vi "Error handler_Init.vi"(0 "reference in":refnum<class "Error handler.lvclass"> caption="This control should only be used when\na sub class is inheriting this class", 3 "LoadFPOnError":bool, 5 "Error In":errorcluster, 6 "Name":string, 8 "Testing":bool) -> (14 "reference out":refnum<class "Error handler.lvclass"> caption="This indicator should only be used when\na sub class is inheriting this class", 19 "Error Out":errorcluster)   [LabVIEW 2019, in "Error handler.lvclass"]
uses:
  Error handler.lvclass
  <vilib>/Utility/sysdir.llb/System Directory Type.ctl
  ErrorLogFile_class/ErrorLogFile.lvclass
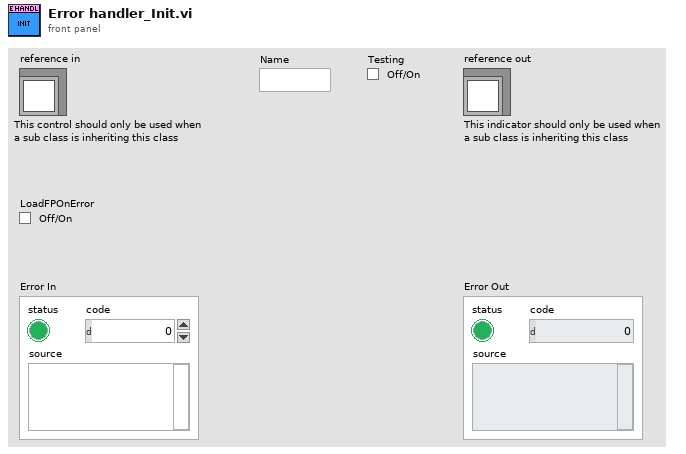
[diagram p1: front panel]
types:
  T1 = typedef "Error handler.lvclass/ObjectAttributes.ctl" = cluster{"ErrorBroadcastEvent":refnum<user-event>, "LoadFPOnError":bool, "ErrorLogFile":refnum<class "ErrorLogFile.lvclass">, "Testing":bool, "Name":string}
  T2 = typedef "System Directory Type.ctl" = i32
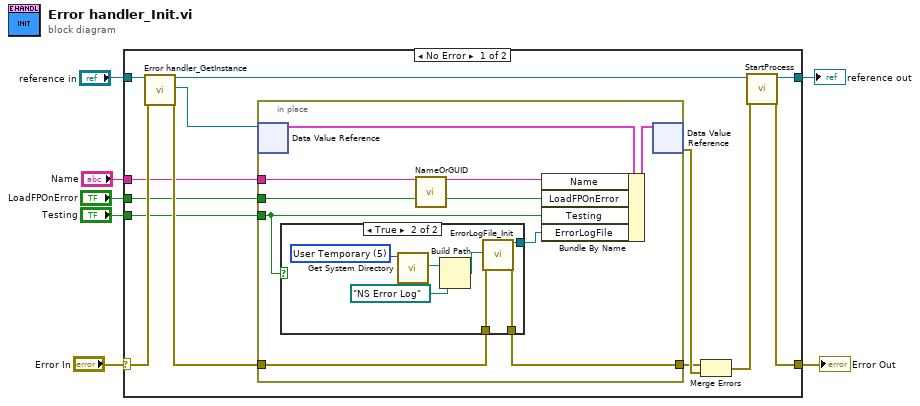
[diagram p0: block diagram]
diagram:
  n1 = case shown="No Error" "Error In" {
    selector: "Error In" -> [w19 w39]
    tunnel: [w11 w39] -> w6
    tunnel: "reference in" -> [w18 w38]
    tunnel: [w13 w38] -> w4
    tunnel: "LoadFPOnError" -> [w10 _]
    tunnel: "Testing" -> [w9 _]
    tunnel: "Name" -> [w8 _]
    frame No Error {
      n2 = call "Error handler_GetInstance.vi"("reference in"=w18, "error in"=w19) -> ("reference out"=w14:refnum<class "Error handler.lvclass">, "DVRRefOut"=w17:refnum<data-value>, "error out"=w16:errorcluster)  [unwired: 13 in, 2 out]
      n3 = in-place {
        in-place-border: w16 -> [w23]
        in-place-border: [w24] -> w15
        in-place-border: w10 -> [w27]
        in-place-border: w9 -> [w26]
        in-place-border: w8 -> [w22]
        n4 = in-place-dvr #1(w17) -> (w28:T1)  [unwired: 1 out]
        n5 = case shown="True" w26 {
          tunnel: [_ w34] -> w25
          tunnel: w23 -> [w30 w33]
          tunnel: [w30 w32] -> w24
          frame False {
          }
          frame True {
            w37 = T2 5 items=["User Home"=0, "User Desktop"=1, "User Documents"=2, "User Application Data"=3, "User Preferences"=4, "User Temporary"=5, "Public Documents"=6, "Public Application Data"=7, "Public Preferences"=8, "Public Cache"=13, "System Core Libraries"=9, "System Installed Libraries"=10, "Application Files"=11, "Boot Volume Root"=12] ("system directory type")
            n6 = call <vilib>:"Get System Directory.vi"("system directory type"=w37) -> ("system directory"=w36:path)  [unwired: 10 in]
            n7 = Build Path(base path=w36, name or relative path=path "NS Error Log") -> (appended path=w31:path)
            n8 = call "ErrorLogFile_Init.vi"("Folder"=w31, "Error In"=w33) -> ("object out"=w34:refnum<class "ErrorLogFile.lvclass">, "Error Out"=w32:errorcluster)  [unwired: 16 in]
          }
        }
        n9 = call "NameOrGUID.vi"("Name"=w22) -> ("NameOrGUID"=w21:string)  [unwired: 18 in]
        n10 = Bundle By Name(cluster=w28, "Name"=w21, "LoadFPOnError"=w27, "Testing"=w26, "ErrorLogFile"=w25) -> (w29:T1)
        n11 = in-place-dvr #1(w29) -> (w20:errorcluster)  [unwired: 1 out]
      }
      n12 = Merge Errors(w15, w20) -> (w12:errorcluster)
      n13 = call "StartProcess.vi"("reference in"=w14, "Error In"=w12) -> ("reference out"=w13:refnum<class "Error handler.lvclass">, "Error Out"=w11:errorcluster)  [unwired: 14 in, 2 out]
    }
    frame Error {
    }
  }
  "Error Out" <- w6
  "reference out" <- w4
